vi "Log Timer.vi"(9 "minutes to log":dbl, 10 "Log?":bool, 11 "Log Start (s)":dbl caption="Present (s)") -> (3 "Time has Elapsed":bool)   [LabVIEW 2013]
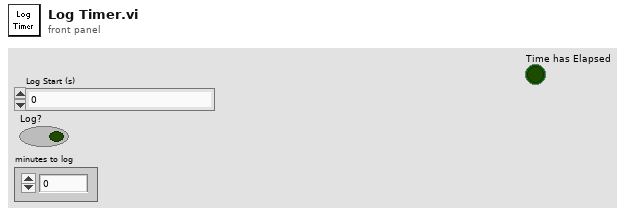
[diagram p1: front panel]
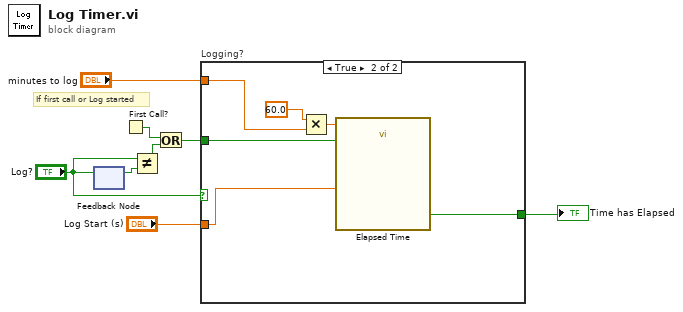
[diagram p0: block diagram]
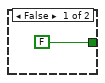
[diagram p2: hidden frame]
diagram:
  # "If first call or Log started"
  n1 = feedback #1() -> (w8:bool)  [unwired: 1 in]
  n2 = feedback-in #1("Log?") -> ()
  n3 = First Call?() -> (First Call?: T/F=w6:bool)
  n4 = Not Equal?(x="Log?", y=w8) -> (x != y?=w5:bool)
  n5 = Or(x=w6, y=w5) -> (x .or. y?=w4:bool)
  n6 = case "Logging?" shown="True" "Log?" {
    tunnel: w4 -> [_ w13]
    tunnel: "minutes to log" -> [_ w12]
    tunnel: "Log Start (s)" -> [_ w10]
    tunnel: [FALSE ("Time has Elapsed") w11] -> w1
    frame False {
    }
    frame True {
      n7 = Multiply(x=60.0 ("y"), y=w12) -> (x*y=w15:dbl)
      n8 = call "Elapsed Time"("Time Target (s)"=w15, "Reset"=w13, "Set Start Time (s)"=w10) -> ("Time has Elapsed"=w11:bool)  [unwired: 9 in, 7 out]
    }
  }
  "Time has Elapsed" <- w1
